vi "Build Inheritance Map.vi"(9 "Subclass Name":string, 10 "Base Class Name":string, 11 "Inheritance Map":T1) -> (3 "Augmented Inheritance Map":T1)   [LabVIEW 2013]
uses:
  <userlib>/ICON Technologies/ICON Maps/lvlib/Map.ctl
  <userlib>/ICON Technologies/ICON Maps/lvlib/_Polymorphic Instances/Map_Value_Variant.vi
  <userlib>/ICON Technologies/ICON Maps/lvlib/_Polymorphic Instances/Map_Insert_Variant.vi
  <userlib>/ICON Technologies/ICON Maps/ICON Maps.lvlib
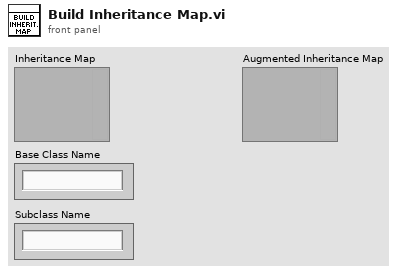
[diagram p1: front panel]
types:
  T1 = typedef "ICON Maps.lvlib/Map.ctl" = variant
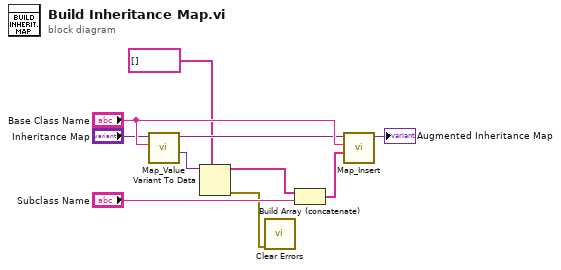
[diagram p0: block diagram]
diagram:
  n1 = call-poly <userlib>:"Map_Value.vi"("Key"="Base Class Name", "Map In"="Inheritance Map") -> ("Value"=w4:variant, "Map Out"=w8:T1)  [unwired: 8 in]
  n2 = Variant To Data(type=string[] [] ("value 2"), Variant=w4) -> (data=w5:string[], error out=w1:errorcluster)  [unwired: 1 in]
  n3 = call <vilib>:"Clear Errors.vi"("error in (no error)"=w1) -> ()  [unwired: 6 in, 1 out]
  n4 = Build Array (concatenate)(w5, "Subclass Name") -> (w6:string[])
  n5 = call-poly <userlib>:"Map_Insert.vi"("Value"=w6, "Key"="Base Class Name", "Map In"=w8) -> ("Map Out"=→"Augmented Inheritance Map":T1)  [unwired: 8 in]
